vi "LM35_Basic.vi"() -> ()   [LabVIEW 2021]
uses:
  <vilib>/Utility/error.llb/DialogType.ctl
  <vilib>/Instr/_visa.llb/VISA Configure Serial Port (Instr).vi
panel:
  out "read buffer":string="\r\n"
  in  "STOP":bool
  in  "VISA resource name":refnum<visa-resource-name>="COM4"
  out "Waveform Chart":cluster{dbl}(graph)
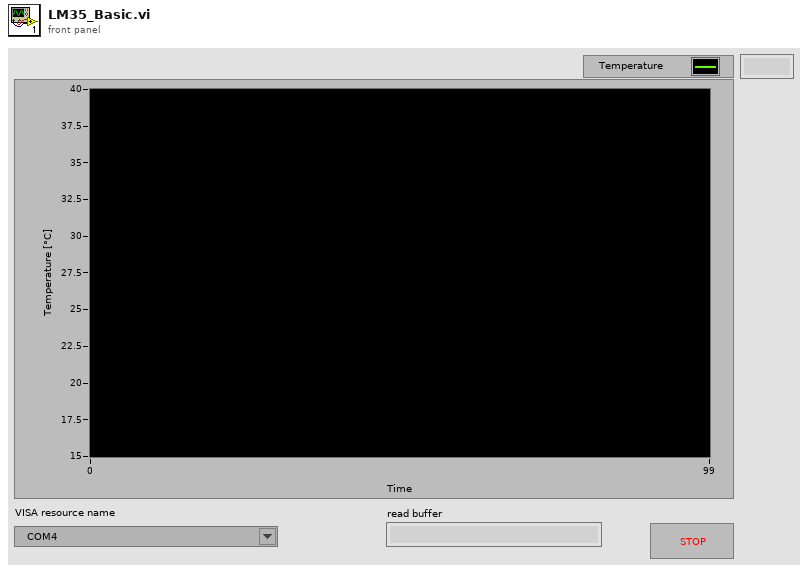
[diagram p1: front panel]
types:
  T1 = typedef "DialogType.ctl" = u16
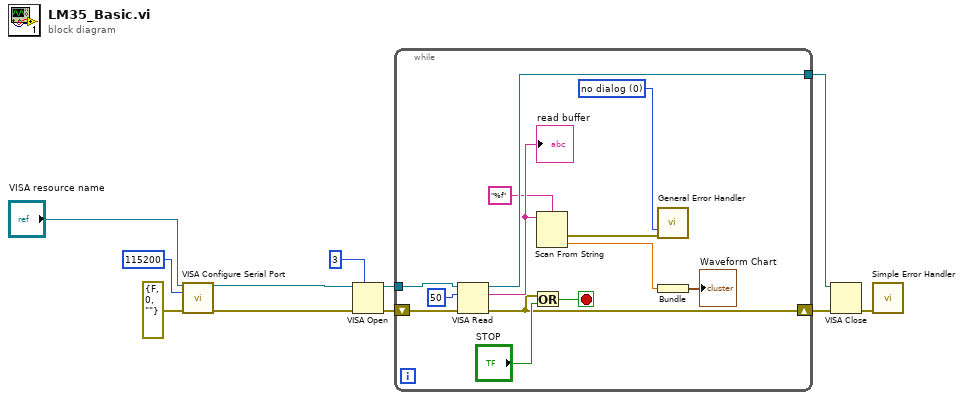
[diagram p0: block diagram]
diagram:
  n1 = call-poly "VISA Configure Serial Port"("VISA resource name"="VISA resource name", "baud rate (9600)"=u32 115200, "error in (no error)"=errorcluster {"status"=FALSE, "code"=0, "source"=""}) -> ("VISA resource name out"=w9:refnum<visa-resource-name>, "error out"=w10:errorcluster)  [unwired: 11 in]
  n2 = VISA Open(timeout (0)=u32 3 ("VISA Open timeout (0)"), error in (no error)=w10, VISA resource name=w9) -> (VISA resource name=w2:refnum<visa-resource-name>, error out=w1:errorcluster)  [unwired: 2 in]
  n3 = while {
    tunnel: w2 -> [w24]
    tunnel: [w20] -> w6
    shift-right: [w16] -> w8
    shift-left: w1 -> [w23]
    stop <- w22 stop-if-true
    w14 = T1 0 items=["no dialog", "OK message", "continue or stop message", "OK message + warnings", "continue/stop + warnings"] ("type of dialog (OK msg:1)")
    n4 = VISA Read(VISA resource name=w24, byte count=u32 50, error in (no error)=w23) -> (VISA resource name out=w20:refnum<visa-resource-name>, read buffer=w19:string, error out=w16:errorcluster)  [unwired: 1 out]
    "read buffer" <- w19
    n5 = Or(x=w16, y="STOP") -> (x .or. y?=w22:bool)
    n6 = Scan From String "Scan From String"(format string="%f", input string=w19) -> (error out=w15:errorcluster, output 1=w12:dbl)  [unwired: 3 in, 2 out]
    n7 = call <vilib>:"General Error Handler.vi"("type of dialog (OK msg:1)"=w14, "error in (no error)"=w15) -> ()  [unwired: 9 in, 5 out]
    n8 = Bundle(w12) -> (→"Waveform Chart":cluster{dbl})  [unwired: 1 in]
  }
  n9 = VISA Close(VISA resource name=w6, error in (no error)=w8) -> (error out=w7:errorcluster)
  n10 = call <vilib>:"Simple Error Handler.vi"("error in (no error)"=w7) -> ()  [unwired: 4 in, 5 out]
